vi "Write Libraries.vi"(10 "Libraries":T1, 11 "ProjectItem in":refnum<class "Search.lvclass">) -> (3 "ProjectItem out":refnum<class "Search.lvclass">)   [LabVIEW 2016, in "Search.lvclass"]
uses:
  Search.lvclass
  Search.lvclass/Search.ctl
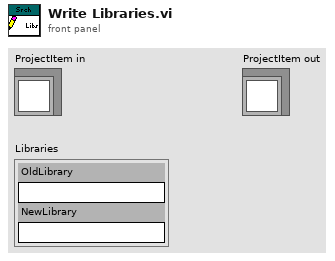
[diagram p1: front panel]
types:
  T1 = cluster{"OldLibrary":string, "NewLibrary":string}
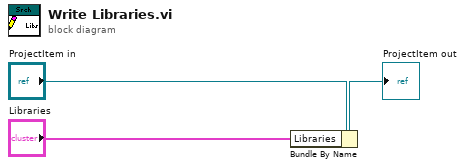
[diagram p0: block diagram]
diagram:
  n1 = Bundle By Name(cluster="ProjectItem in", "Libraries"="Libraries") -> (→"ProjectItem out":refnum<class "Search.lvclass">)
